vi "Response.vi"(9 "rsp":u32) -> (1 "error":string)   [LabVIEW 2019, in "FINS TCP.lvlib"]
uses:
  FINS TCP.lvlib
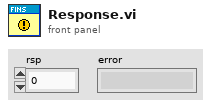
[diagram p1: front panel]
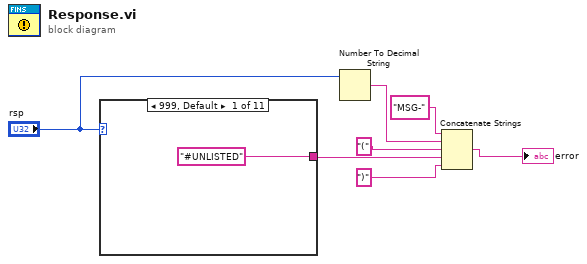
[diagram p0: block diagram]
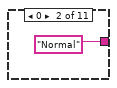
[diagram p2: hidden frame]
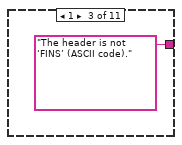
[diagram p3: hidden frame]
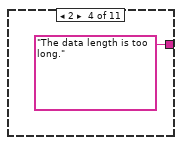
[diagram p4: hidden frame]
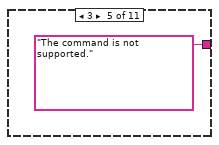
[diagram p5: hidden frame]
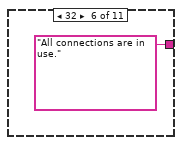
[diagram p6: hidden frame]
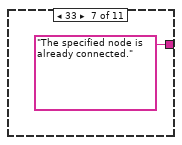
[diagram p7: hidden frame]
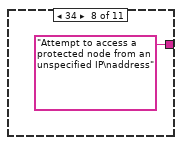
[diagram p8: hidden frame]
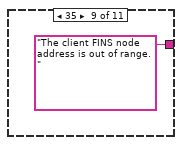
[diagram p9: hidden frame]
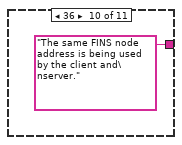
[diagram p10: hidden frame]
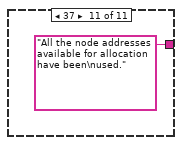
[diagram p11: hidden frame]
diagram:
  n1 = case shown="999, Default" "rsp" {
    tunnel: ["#UNLISTED" "Normal" "The header is not ‘FINS’ (ASCII code)." "The data length is too long." "The command is not supported." "All connections are in use." "The specified node is already connected." "Attempt to access a protected node from an unspecified IP\naddress" "The client FINS node address is out of range." "The same FINS node address is being used by the client and\nserver." "All the node addresses available for allocation have been\nused."] -> w6
    frame 999, Default {
    }
    frame 0 {
    }
    frame 1 {
    }
    frame 2 {
    }
    frame 3 {
    }
    frame 32 {
    }
    frame 33 {
    }
    frame 34 {
    }
    frame 35 {
    }
    frame 36 {
    }
    frame 37 {
    }
  }
  n2 = Number To Decimal String(number="rsp") -> (decimal integer string=w5:string)  [unwired: 1 in]
  n3 = Concatenate Strings("MSG-" ("string"), w5, "(" ("string"), w6, ")" ("string")) -> (→"error":string)
